vi "Create.vi"(8 "error in (no error)":errorcluster) -> (0 "error out":errorcluster, 3 "BL-Extend-Cmd out":refnum<class "BL-Extend-Cmd.lvclass">)   [LabVIEW 2013, in "BL-Extend-Cmd.lvclass"]
uses:
  BL-Extend-Cmd.lvclass
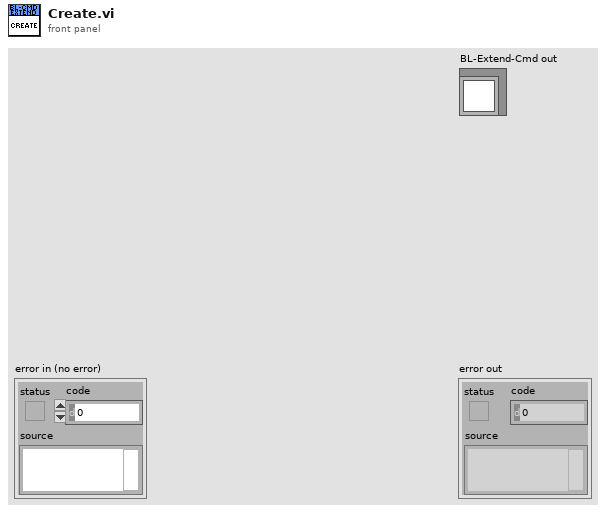
[diagram p1: front panel]
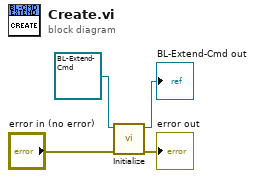
[diagram p0: block diagram]
diagram:
  n1 = call-dynamic "Initialize.vi"("error in (no error)"="error in (no error)", "BL-Extend-Cmd in"=refnum<class "BL-Extend-Cmd.lvclass"> refnum ("BL-Extend-Cmd.lvclass")) -> ("error out"=→"error out":errorcluster, "BL-Extend-Cmd out"=→"BL-Extend-Cmd out":refnum<class "BL-Extend-Cmd.lvclass">)  [unwired: 8 in]
